vi "NFC_Result.vi"(9 "input":string, 10 "return code":i32) -> (1 "Command Sucess":bool, 2 "return_result":string)   [LabVIEW 2017]
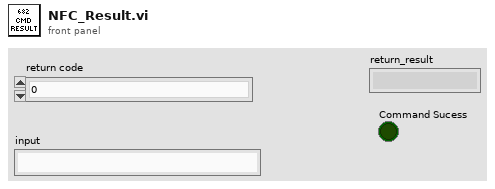
[diagram p1: front panel]
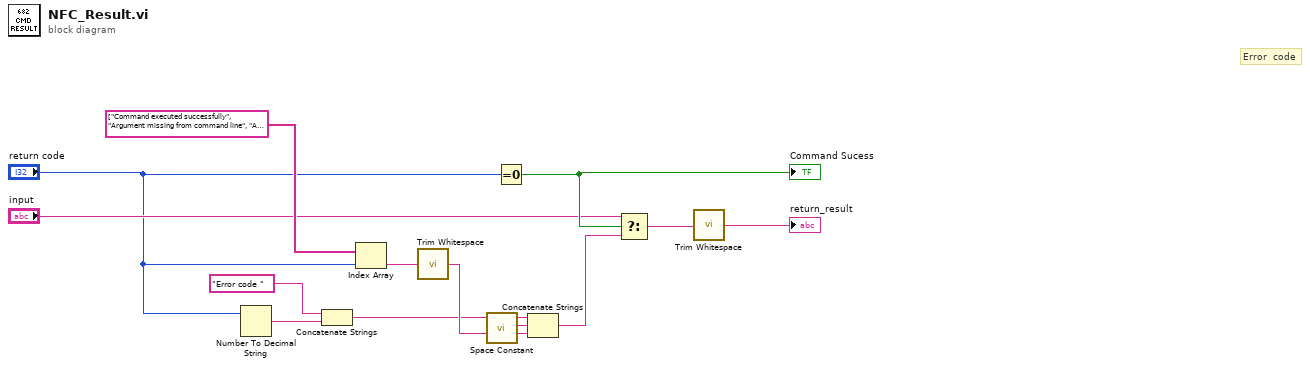
[diagram p0: block diagram]
diagram:
  # "Error  code"
  n1 = Number To Decimal String(number="return code") -> (decimal integer string=w7:string)  [unwired: 1 in]
  n2 = Concatenate Strings("Error code ", w7) -> (w6:string)
  n3 = Index Array(array=string[] ["Command executed successfully", "Argument missing from command line", "An invalid argument wasa provided to command line", "Connection error occurred or no connection", "A message was sent out but did not receive a response in time or there was no response at all\n", "An invalid test parameter was supplied\n", "An invalid test parameter was supplied", "An unknown error has occurred, but details should be provided depending on the test case being run\n"], index="return code") -> (element=w5:string)
  n4 = call <vilib>:"Trim Whitespace.vi"("string"=w5) -> ("trimmed string"=w10:string)  [unwired: 1 in]
  n5 = call <vilib>:"Space Constant.vi"() -> ("String"=w1:string)
  n6 = Equal To 0?(x="return code") -> (x = 0?=w12:bool)
  "Command Sucess" <- w12
  n7 = Concatenate Strings(w6, w1, w10) -> (w4:string)
  n8 = Select(t="input", s=w12, f=w4) -> (s? t:f=w3:string)
  n9 = call <vilib>:"Trim Whitespace.vi"("string"=w3) -> ("trimmed string"=→"return_result":string)  [unwired: 1 in]
